vi "Actor Core.vi"(8 "error in":errorcluster, 11 "Caller B in":refnum<class "Caller B.lvclass">) -> (0 "error out":errorcluster, 3 "Actor out":refnum<class "Actor.lvclass">)   [LabVIEW 2023, in "Caller B.lvlib" / "Caller B.lvclass"]
doc: "(<B>Filename</B>: Actor Framework.lvlib:Actor.lvclass:Actor Core.vi)\n\nReceives messages to the actor, reacts to them, and initiates any error handling that may shut the actor down.\n\nDescendant classes may override this VI to append parallel tasks for the actor to complete while it handles messages. Overrides use the Call Parent Method node."
uses:
  Caller B.lvclass
  c:/dev/_r/4/eng/lv-core/lvpostprocessingd/lv_mc_x86_64/dist_i386/vi.lib/ActorFramework/Actor/Actor.lvclass
  <vilib>/ActorFramework/Actor/Actor.lvclass
  Nested/Nested/Nested.lvclass
  <vilib>/ActorFramework/Actor/Actor.lvclass/Actor.ctl
  <vilib>/ActorFramework/Message Enqueuer/Message Enqueuer.lvclass/Message Enqueuer.ctl
  Caller B.lvclass/Caller B.ctl
  Nested/Nested/Named Value.ctl
  Nested/Nested Messages/Lookup Value Msg/Lookup Value Msg.lvclass/Lookup Value Msg.ctl
  <vilib>/ActorFramework/Message Enqueuer/Init from Existing Queue.vi
  <vilib>/ActorFramework/Message Enqueuer/Enqueue.vi
  <vilib>/ActorFramework/Stop Msg/Stop Msg.lvclass
  c:/dev/_r/4/eng/lv-core/lvpostprocessingd/lv_mc_x86_64/dist_i386/vi.lib/ActorFramework/Message/Message.lvclass
  Nested/Nested Messages/Lookup Value Msg/Lookup Value Msg.lvclass
  Localization.vi
  <vilib>/ActorFramework/Message Priority Queue/Priority Enqueue.vi
  <vilib>/ActorFramework/Message Enqueuer/Message Enqueuer.lvclass
  Parent of Caller B/Parent of Caller B/Parent of Caller B.lvclass
panel:
  out "event log":string
  in  "stop":bool
  in  "lookup golden ratio":bool
  in  "lookup e":bool
  in  "lookup pi":bool
  # "B"
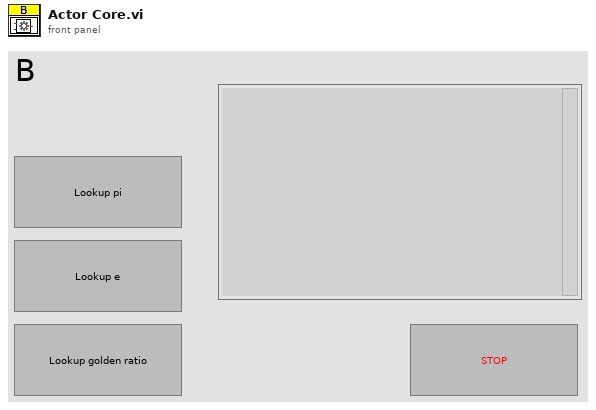
[diagram p1: front panel]
types:
  T1 = typedef "Nested.lvlib/Nested.lvclass/Named Value.ctl" = enum16{"e", "pi", "golden ratio"}
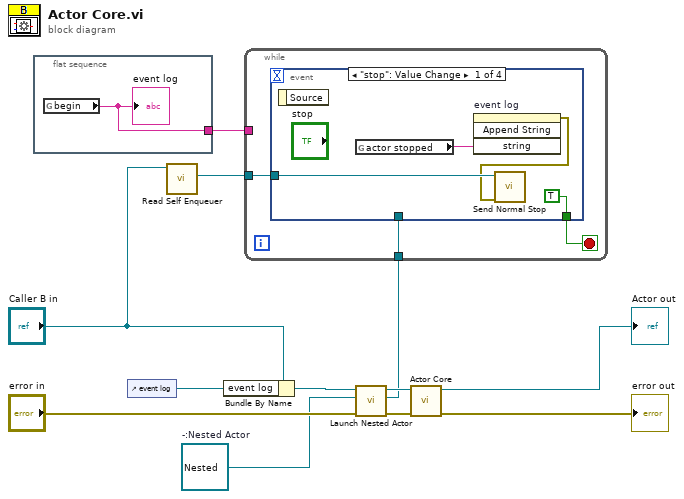
[diagram p0: block diagram]
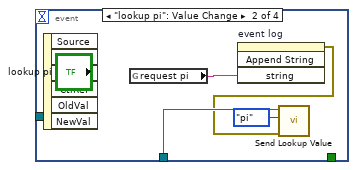
[diagram p2: hidden frame]
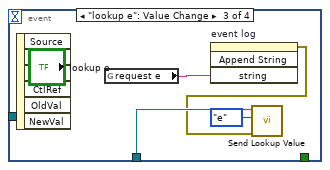
[diagram p3: hidden frame]
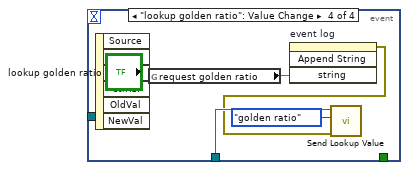
[diagram p4: hidden frame]
diagram:
  w7 = refnum<class "Nested.lvclass"> refnum  # -:Nested Actor
  n1 = flat-sequence {
    tunnel: [w13] -> w1
    frame #0 {
      n2 = global read "Localization.vi" "begin"() -> (w13:string)
      "event log" <- w13
    }
  }
  n3 = control-ref of="event log"() -> (w5:refnum<vi>)
  n4 = call <vilib>:"Read Self Enqueuer.vi"("Actor"="Caller B in") -> ("Self Enqueuer"=w3:refnum<class "Message Enqueuer.lvclass">)  [unwired: 10 in]
  n5 = Bundle By Name(cluster="Caller B in", "event log"=w5) -> (w6:refnum<class "Caller B.lvclass">)
  n6 = call <vilib>:"Launch Nested Actor.vi"("error in (no error)"="error in", "Nested Actor"=w7, "Caller Actor in"=w6) -> ("error out"=w9:errorcluster, "Nested Actor's Enqueuer"=w2:refnum<class "Message Enqueuer.lvclass">, "Caller Actor out"=w10:refnum<class "Caller B.lvclass">)  [unwired: 6 in]
  n7 = while {
    tunnel: w3 -> [w15]
    tunnel: w2 -> [w14]
    tunnel: w1 -> [_]
    stop <- w16 stop-if-true
    n8 = event shown="[0] \"stop\": Value Change" {
      selector: _ -> [_ _ _ _]
      dyn-events: _ -> [_ _ _ _]
      timeout: _ -> [_ _ _ _]
      tunnel: [TRUE _ _ _] -> w16
      tunnel: w15 -> [w19 _ _ _]
      tunnel: w14 -> [_ w24 w28 w32]
      event "stop": Value Change {
        n9 = event-data() -> ()  [unwired: 1 in, 1 out]
        n10 = global read "Localization.vi" "actor stopped"() -> (w18:string)
        n11 = invoke on="event log" class="Str" method="Append String"("string"=w18) -> (error out=w17:errorcluster)  [unwired: 3 in, 3 out]
        n12 = call <vilib>:"Send Normal Stop.vi"("error in (no error)"=w17, "Message Enqueuer"=w19) -> ()  [unwired: 9 in, 1 out]
      }
      event "lookup pi": Value Change {
        n13 = event-data() -> ()  [unwired: 1 in, 6 out]
        n14 = global read "Localization.vi" "request pi"() -> (w22:string)
        n15 = invoke on="event log" class="Str" method="Append String"("string"=w22) -> (error out=w21:errorcluster)  [unwired: 3 in, 3 out]
        n16 = call "Send Lookup Value.vi"("error in (no error)"=w21, "named value"=Named_Value."pi", "Message Enqueuer"=w24) -> ()  [unwired: 7 in, 2 out]
      }
      event "lookup e": Value Change {
        n17 = event-data() -> ()  [unwired: 1 in, 6 out]
        n18 = global read "Localization.vi" "request e"() -> (w26:string)
        n19 = invoke on="event log" class="Str" method="Append String"("string"=w26) -> (error out=w25:errorcluster)  [unwired: 3 in, 3 out]
        n20 = call "Send Lookup Value.vi"("error in (no error)"=w25, "named value"=Named_Value."e", "Message Enqueuer"=w28) -> ()  [unwired: 7 in, 2 out]
      }
      event "lookup golden ratio": Value Change {
        n21 = event-data() -> ()  [unwired: 1 in, 6 out]
        n22 = global read "Localization.vi" "request golden ratio"() -> (w30:string)
        n23 = invoke on="event log" class="Str" method="Append String"("string"=w30) -> (error out=w29:errorcluster)  [unwired: 3 in, 3 out]
        n24 = call "Send Lookup Value.vi"("error in (no error)"=w29, "named value"=Named_Value."golden ratio", "Message Enqueuer"=w32) -> ()  [unwired: 7 in, 2 out]
      }
    }
  }
  n25 = call-parent "Actor Core.vi"("error in"=w9, "Actor in"=w10) -> ("error out"=→"error out":errorcluster, "Actor out"=→"Actor out":refnum<class "Actor.lvclass">)  [unwired: 8 in]
